vi "CorrectResponse.vi"(8 "error in (no error)":errorcluster, 11 "TrialBasedExperiment in":refnum<class "WhiteNoiseOrientationDetection.lvclass">) -> (0 "error out":errorcluster, 3 "TrialBasedExperiment out":refnum<class "WhiteNoiseOrientationDetection.lvclass">)   [LabVIEW 2012, in "WhiteNoiseOrientationDetection.lvclass"]
uses:
  WhiteNoiseOrientationDetection.lvclass
  Trial Based Experiment Statechart/MatlabExperiment/MatlabExperiment.lvclass
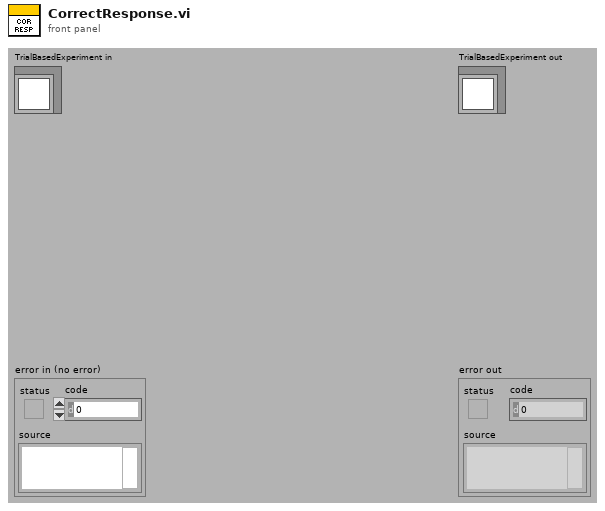
[diagram p1: front panel]
types:
  T1 = cluster{"Intertrial":dbl, "AcquireFixation":dbl, "HoldFixation":dbl, "DelayPeriod":dbl, "ResponsePeriod":dbl}
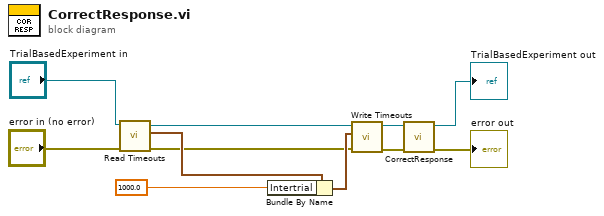
[diagram p0: block diagram]
diagram:
  n1 = call-dynamic "Read Timeouts.vi"("error in (no error)"="error in (no error)", "TrialBasedExperiment in"="TrialBasedExperiment in") -> ("error out"=w8:errorcluster, "Timeouts"=w11:T1, "TrialBasedExperiment out"=w9:refnum<class "WhiteNoiseOrientationDetection.lvclass">)  [unwired: 7 in]
  n2 = Bundle By Name(cluster=w11, "Intertrial"=1000.0) -> (w10:T1)
  n3 = call-dynamic "Write Timeouts.vi"("error in (no error)"=w8, "Timeouts"=w10, "TrialBasedExperiment in"=w9) -> ("error out"=w4:errorcluster, "TrialBasedExperiment out"=w5:refnum<class "WhiteNoiseOrientationDetection.lvclass">)  [unwired: 7 in]
  n4 = call-parent "CorrectResponse.vi"("error in (no error)"=w4, "TrialBasedExperiment in"=w5) -> ("error out"=→"error out":errorcluster, "TrialBasedExperiment out"=→"TrialBasedExperiment out":refnum<class "WhiteNoiseOrientationDetection.lvclass">)  [unwired: 8 in]
